vi "CoilsToNumbers.vi"(10 "Coils":bool[](array[boolean])) -> (2 "16bitValues":u16[](array[numeric]))   [LabVIEW 2018]
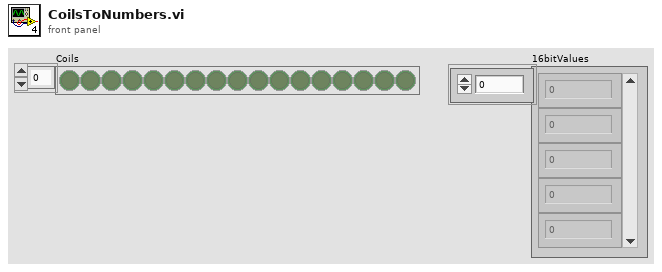
[diagram p1: front panel]
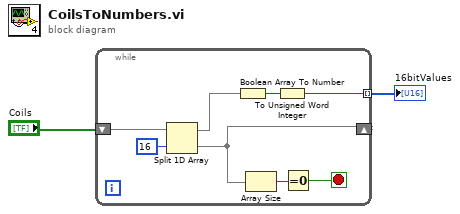
[diagram p0: block diagram]
diagram:
  n1 = while {
    shift-right: [w6] -> _
    shift-left: "Coils" -> [w10]
    tunnel: [w3] -> w1 mode=indexing
    stop <- w4 stop-if-true
    n2 = Split 1D Array(array=w10, index=16) -> (first subarray=w8:bool[], second subarray=w6:bool[])
    n3 = Boolean Array To Number(Boolean array=w8) -> (number=w7:u32)
    n4 = Array Size(array=w6) -> (size(s)=w5:i32)
    n5 = To Unsigned Word Integer(number=w7) -> (unsigned 16bit integer=w3:u16)
    n6 = Equal To 0?(x=w5) -> (x = 0?=w4:bool)
  }
  "16bitValues" <- w1
